vi "nanomsg_poll.vi"   [LabVIEW 2014, in "nanomsg.lvlib" / "nanomsg_socket.lvclass"]
uses:
  nanomsg_socket.lvclass
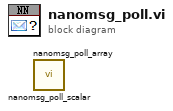
[diagram p0: block diagram]
diagram:
  n1 = call "nanomsg_poll_scalar.vi"() -> ()  [unwired: 4 in, 4 out]
  n2 = call "nanomsg_poll_array.vi"() -> ()  [unwired: 4 in, 4 out]
